vi "test Get Attribute as JSON.vi"(11 "Test Case In":refnum<class "Test Config From EXCEL.lvclass">) -> (0 "error out":errorcluster, 3 "Test Case Out":refnum<class "Test Config From EXCEL.lvclass">)   [LabVIEW 2024, in "Test Config From EXCEL.lvclass"]
uses:
  Test Config From EXCEL.lvclass
  C:/Program Files/National Instruments/LabVIEW 2025/vi.lib/Astemes/LUnit/Test Case.lvclass
  Config from EXCEL/Config from EXCEL.lvclass
  <vilib>/Astemes/LUnit/Test Case.lvclass/Test Case.ctl
  <vilib>/Astemes/LUnit/Append Fail Result.vi
  <vilib>/Astemes/LUnit/Append Pass Result.vi
  <vilib>/Astemes/LUnit/Run In UI.vi
  <vilib>/Utility/error.llb/Clear Errors.vi
  <vilib>/JDP Science/JSONtext/JSONtext.lvlib
  <vilib>/Astemes/LUnit/Test Case.lvclass
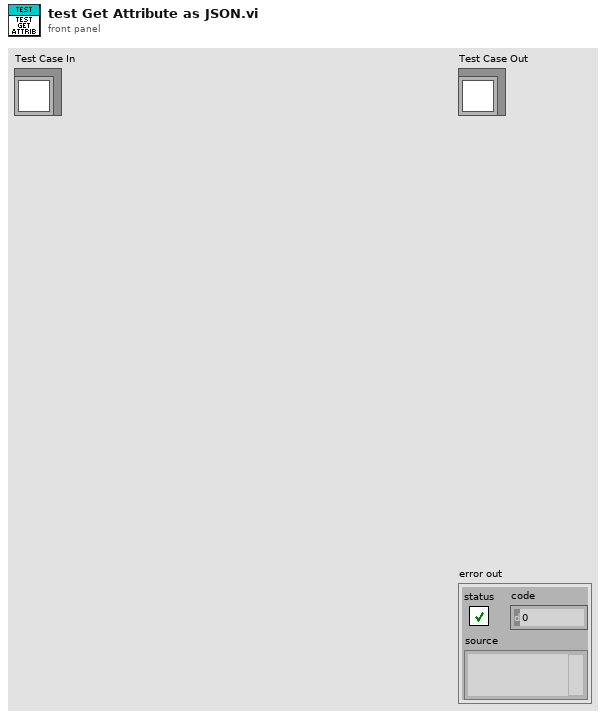
[diagram p1: front panel]
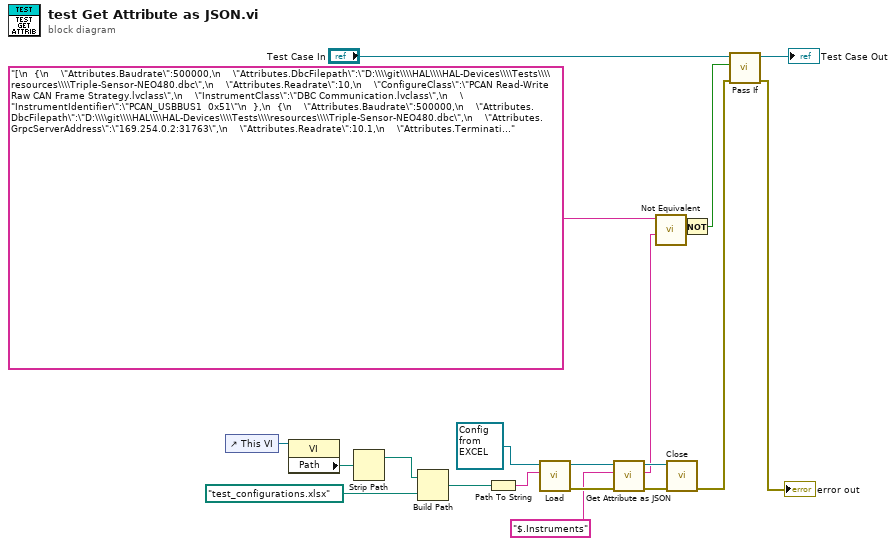
[diagram p0: block diagram]
diagram:
  n1 = control-ref of="This VI"() -> (w14:refnum<vi>)
  n2 = property class="VI"(reference=w14) -> ("Path"=w13:path)  [unwired: 1 in, 2 out]
  n3 = Strip Path(path=w13) -> (stripped path=w11:path)  [unwired: 1 out]
  n4 = Build Path(base path=w11, name or relative path=path "test_configurations.xlsx") -> (appended path=w12:path)
  n5 = Path To String(path=w12) -> (string=w15:string)
  n6 = call-dynamic "Load.vi"("Source"=w15, "Config from EXCEL in"=refnum<class "Config from EXCEL.lvclass"> refnum ("Config from EXCEL.lvclass")) -> ("error out"=w8:errorcluster, "Config from EXCEL out"=w9:refnum<class "Config from EXCEL.lvclass">)  [unwired: 8 in]
  n7 = call-dynamic "Get Attribute as JSON.vi"("error in"=w8, "Attribute"="$.Instruments", "Config from EXCEL in"=w9) -> ("error out"=w6:errorcluster, "<JSON>"=w4:string, "Config from EXCEL out"=w5:refnum<class "Config from EXCEL.lvclass">)  [unwired: 6 in]
  n8 = call <vilib>:"Not Equivalent.vi"("Other JSON"=w4, "JSON"="[\n  {\n    \"Attributes.Baudrate\":500000,\n    \"Attributes.DbcFilepath\":\"D:\\\\git\\\\HAL\\\\HAL-Devices\\\\Tests\\\\resources\\\\Triple-Sensor-NEO480.dbc\",\n    \"Attributes.Readrate\":10,\n    \"ConfigureClass\":\"PCAN Read-Write Raw CAN Frame Strategy.lvclass\",\n    \"InstrumentClass\":\"DBC Communication.lvclass\",\n    \"InstrumentIdentifier\":\"PCAN_USBBUS1  0x51\"\n  },\n  {\n    \"Attributes.Baudrate\":500000,\n    \"Attributes.DbcFilepath\":\"D:\\\\git\\\\HAL\\\\HAL-Devices\\\\Tests\\\\resources\\\\Triple-Sensor-NEO480.dbc\",\n    \"Attributes.GrpcServerAddress\":\"169.254.0.2:31763\",\n    \"Attributes.Readrate\":10.1,\n    \"Attributes.Termination\":1,\n    \"ConfigureClass\":\"gRPC XNET Read Raw CAN Frame Strategy.lvclass\",\n    \"InstrumentClass\":\"DBC Communication.lvclass\",\n    \"InstrumentIdentifier\":\"CAN1\"\n  }\n]" ("<JSON>")) -> ("Not Equivalent"=w2:bool)  [unwired: 8 in]
  n9 = call-dynamic "Close.vi"("error in"=w6, "Config from EXCEL in"=w5) -> ("error out"=w10:errorcluster)  [unwired: 8 in, 1 out]
  n10 = Not(x=w2) -> (.not. x?=w1:bool)
  n11 = call <vilib>:"Pass If.vi"("error in (no error)"=w10, "Pass?"=w1, "LUnit Test Case In"="Test Case In") -> ("error out"=→"error out":errorcluster, "LUnit Test Case Out"=→"Test Case Out":refnum<class "Test Config From EXCEL.lvclass">)  [unwired: 7 in]
